vi "Read End-of-File.vi"(8 "Error In":errorcluster, 11 "Channel In":refnum<class "Channel.lvclass">) -> (0 "Error Out":errorcluster, 2 "End-of-File?":bool, 3 "Channel Out":refnum<class "Channel.lvclass">)   [LabVIEW 2018, in "Toolkit.lvlib" / "Channel.lvclass"]
uses:
  Channel.lvclass
  Channel.lvclass/Channel.ctl
  Session/Session.lvclass/Session.ctl
  SSH/SSH.lvclass/SSH.ctl
  Session/Session.lvclass
  Toolkit.lvlib
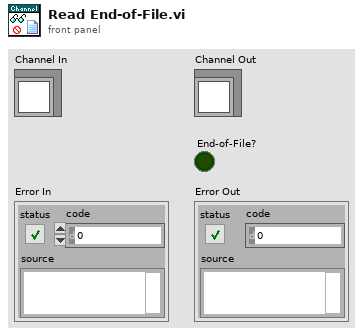
[diagram p1: front panel]
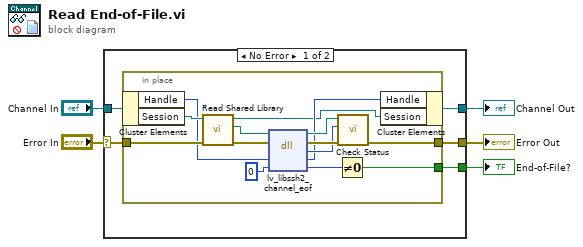
[diagram p0: block diagram]
diagram:
  n1 = case shown="No Error" "Error In" {
    selector: "Error In" -> [w8 w26]
    tunnel: [w7 w26] -> w4
    tunnel: "Channel In" -> [w10 w25]
    tunnel: [w9 w25] -> w2
    tunnel: [w6 _] -> w1
    frame No Error {
      n2 = in-place {
        in-place-border: w8 -> [w21]
        in-place-border: [w17] -> w7
        in-place-border: [w11] -> w6
        n3 = in-place-cluster #1(w10) -> ("Handle"=w16:u64, "Session"=w24:refnum<class "Session.lvclass">)
        n4 = call "Read Shared Library.vi"("Error In"=w21, "Session In"=w24) -> ("Erorr Out"=w22:errorcluster, "libssh2lv Shared Library"=w23:path, "Session Out"=w14:refnum<class "Session.lvclass">)  [unwired: 7 in]
        n5 = dll-call lib="libssh2lv.*" fn="lv_libssh2_channel_eof"(path in=w23, error in=w22, "handle"=w16, "eof"=0) -> (path out=w19:path, error out=w20:errorcluster, "status"=w18:i32, "handle"=w15:u64, "eof"=w12:i32)  [unwired: 1 in]
        n6 = Not Equal To 0?(x=w12) -> (x != 0?=w11:bool)
        n7 = call "Check Status.vi"("Error In"=w20, "Status"=w18, "lv-libssh2 Shared Library In"=w19) -> ("Error Out"=w17:errorcluster)  [unwired: 7 in, 1 out]
        n8 = in-place-cluster #1("Handle"=w15, "Session"=w14) -> (w9:refnum<class "Channel.lvclass">)
      }
    }
    frame Error {
    }
  }
  "Error Out" <- w4
  "Channel Out" <- w2
  "End-of-File?" <- w1
